vi "ASCto16进制字符串.vi"(1 "ASC":string) -> (0 "16进制字符串":string)   [LabVIEW 2014]
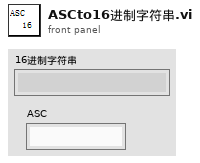
[diagram p1: front panel]
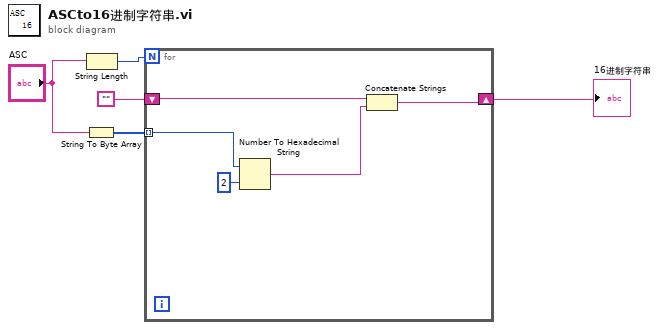
[diagram p0: block diagram]
diagram:
  n1 = String To Byte Array(string="ASC") -> (unsigned byte array=w3:u8[])
  n2 = String Length(string="ASC") -> (length=w5:i32)
  n3 = for {
    N: w5 -> [_]
    tunnel: w3 -> [w10] mode=indexing
    shift-right: [w6] -> w1
    shift-left: "" -> [w8]
    n4 = Number To Hexadecimal String(1:i16 2 ("宽度(-)"), 2:w10) -> (0:w7:string)
    n5 = Concatenate Strings(w8, w7) -> (w6:string)
  }
  "16进制字符串" <- w1
